vi "Test Method 3.vi"(8 "error in (no error)":errorcluster, 11 "Test Case In":refnum<class "LMock Pure Test Case 7.lvclass">) -> (0 "error out":errorcluster, 3 "Test Case Out":refnum<class "LMock Pure Test Case 7.lvclass">)   [LabVIEW 2020, in "LMock Pure Test Case 7.lvclass"]
uses:
  LMock Pure Test Case 7.lvclass
  C:/Program Files (x86)/National Instruments/LabVIEW 2020/vi.lib/Astemes/LUnit/Test Case.lvclass
  Test Interface Pure Mock/Test Interface Pure Mock.lvclass
  C:/Program Files (x86)/National Instruments/LabVIEW 2020/vi.lib/Astemes/LMock/Mock.lvclass
  LMock Pure Test Case 7.lvclass/LMock Pure Test Case 7.ctl
  <vilib>/Astemes/LMock/LMock Verifier.lvclass
  <vilib>/Astemes/LMock/Identical Inputs Comparator.lvclass
  <vilib>/Astemes/LMock/One.lvclass
  C:/Program Files (x86)/National Instruments/LabVIEW 2020/vi.lib/Astemes/LMock/Pure Mock.lvclass
  C:/git/astemes-lmock/sandbox/Benchmark/Test Interface Pure Mock/Test Interface Pure Mock.lvclass
  C:/git/astemes-lmock/sandbox/Benchmark/Test Interface/Test Interface.lvclass
  C:/Program Files (x86)/National Instruments/LabVIEW 2020/vi.lib/Astemes/LUnit/LUnit Runnable.lvclass
  C:/git/astemes-lmock/sandbox/Benchmark/LMock Pure Test Case 7/LMock Pure Test Case 7.lvclass
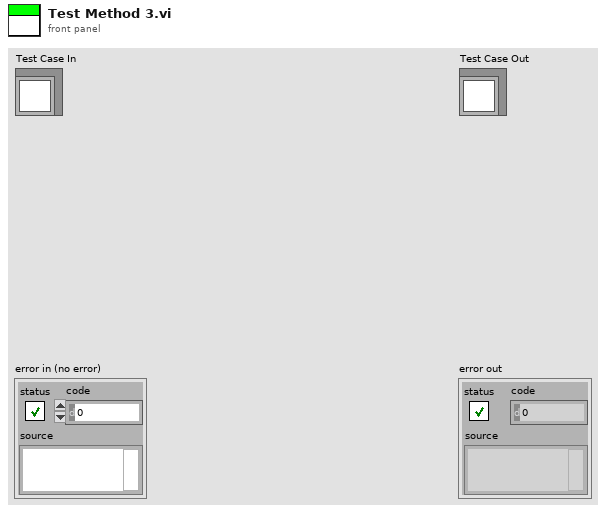
[diagram p1: front panel]
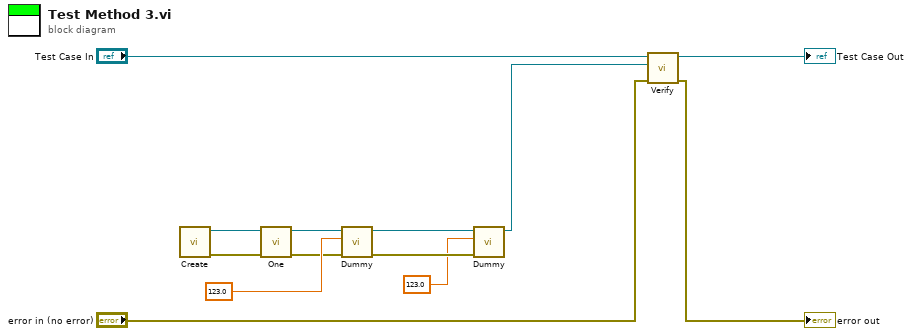
[diagram p0: block diagram]
diagram:
  n1 = call "Create.vi"() -> ("error out"=w9:errorcluster, "Test Interface Pure Mock Out"=w6:refnum<class "Test Interface Pure Mock.lvclass">)  [unwired: 10 in]
  n2 = call <vilib>:"One.vi"("error in (no error)"=w9, "Mock in"=w6) -> ("error out"=w7:errorcluster, "Mock out"=w5:refnum<class "Test Interface Pure Mock.lvclass">)  [unwired: 8 in]
  n3 = call-dynamic "Dummy.vi"("error in (no error)"=w7, "Numeric"=123.0, "Test Interface in"=w5) -> ("error out"=w3:errorcluster, "Test Interface out"=w4:refnum<class "Test Interface Pure Mock.lvclass">)  [unwired: 6 in, 1 out]
  n4 = call-dynamic "Dummy.vi"("error in (no error)"=w3, "Numeric"=123.0, "Test Interface in"=w4) -> ("Test Interface out"=w1:refnum<class "Test Interface Pure Mock.lvclass">)  [unwired: 6 in, 2 out]
  n5 = call-poly <vilib>:"Verify.vi"("error in (no error)"="error in (no error)", "Mock"=w1, "LUnit Test Case In"="Test Case In") -> ("error out"=→"error out":errorcluster, "LUnit Test Case Out"=→"Test Case Out":refnum<class "LMock Pure Test Case 7.lvclass">)  [unwired: 7 in]
